vi "Set Default Headers.vi"(8 "error in (no error)":errorcluster, 11 "Response in":refnum<class "Response.lvclass">) -> (0 "error out":errorcluster, 3 "Response out":refnum<class "Response.lvclass">)   [LabVIEW 2023, in "Response.lvclass"]
uses:
  Response.lvclass
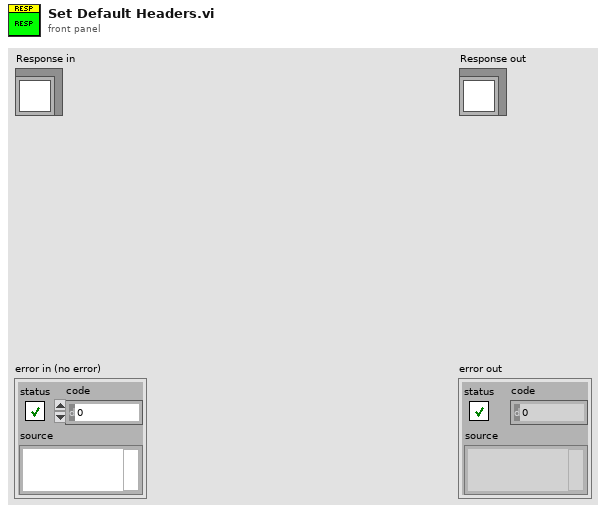
[diagram p1: front panel]
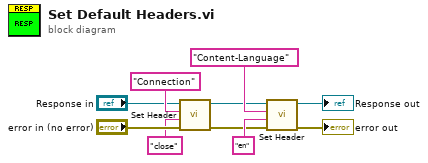
[diagram p0: block diagram]
diagram:
  n1 = call "Set Header.vi"("error in (no error)"="error in (no error)", "Value"="close" ("Header"), "Header"="Connection", "Response in"="Response in") -> ("error out"=w8:errorcluster, "Response out"=w7:refnum<class "Response.lvclass">)  [unwired: 5 in, 1 out]
  n2 = call "Set Header.vi"("error in (no error)"=w8, "Value"="en" ("Header"), "Header"="Content-Language", "Response in"=w7) -> ("error out"=→"error out":errorcluster, "Response out"=→"Response out":refnum<class "Response.lvclass">)  [unwired: 5 in, 1 out]
